vi "Stage Printing Loop.vi"(11 "Stage Actor.lvlib:Stage.lvclass":refnum<class "Stage.lvclass">) -> ()   [LabVIEW 2018, in "Stage Actor.lvlib" / "Stage.lvclass"]
uses:
  Stage.lvclass
  C:/Program Files (x86)/National Instruments/LabVIEW 2018/vi.lib/MGI/Panel Manager/Panel Actor/Panel Actor/Panel Actor.lvclass
  Stage.lvclass/Stage.ctl
  <instrlib>/Zaber A Series/Public/Action-Status/Streaming/Set Stream Speed and Acceleration (FW7).vi
  <instrlib>/Zaber A Series/Public/Action-Status/Streaming/Stream Line (FW7).vi
  <instrlib>/Zaber A Series/Zaber A Series.lvlib
  <vilib>/MGI/Panel Manager/Panel Actor/Panel Actor/Panel Actor.lvclass
panel:
  out "Stop":bool
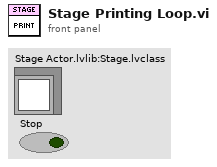
[diagram p1: front panel]
types:
  T1 = cluster{"Print Data":cluster{"XYZ":dbl[][], "Theta Phi":dbl[][], "Current Tool":i16[], "Speed":dbl[], "Feeder State":bool[]}, "Task":string}
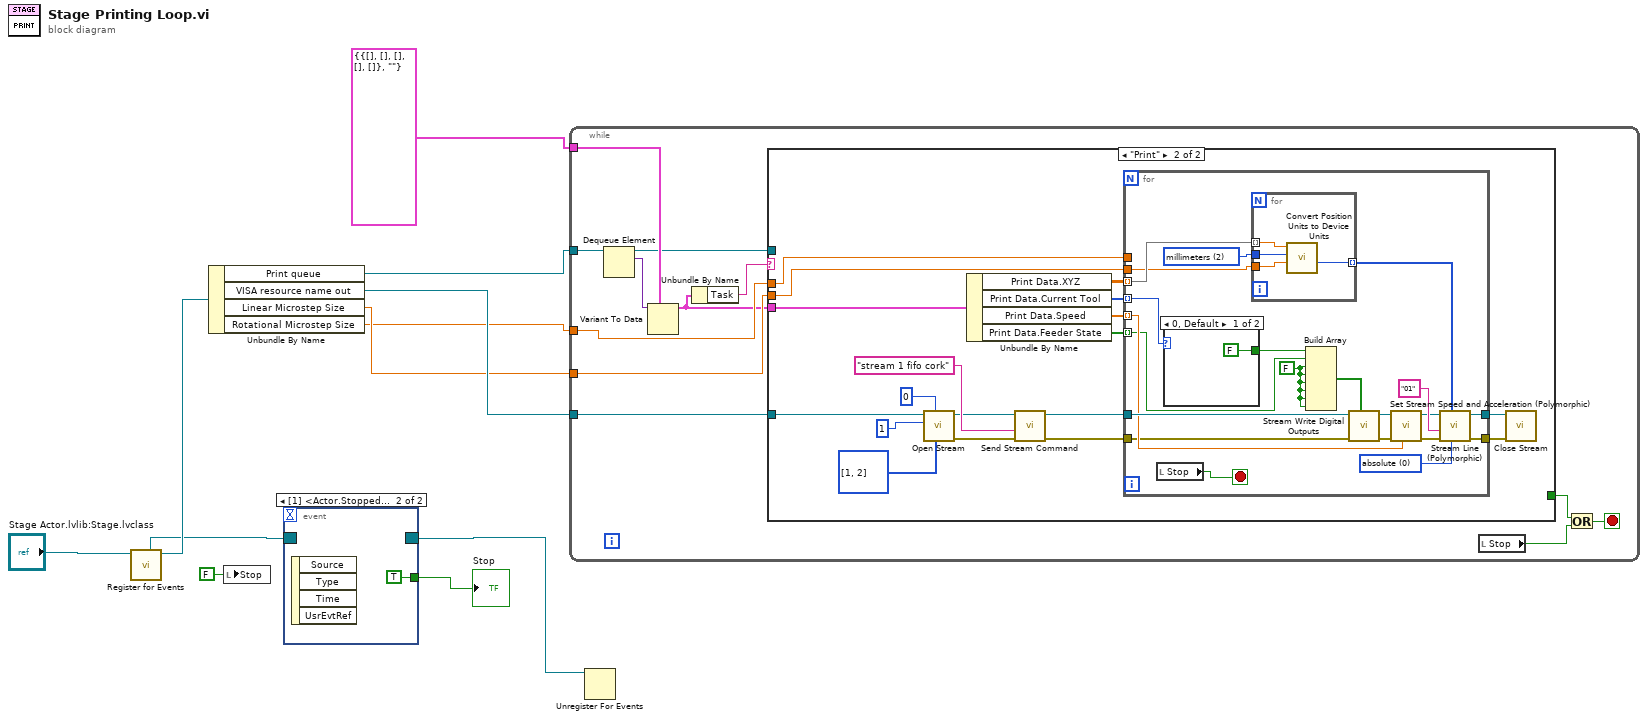
[diagram p0: block diagram]
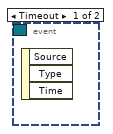
[diagram p2: hidden frame]
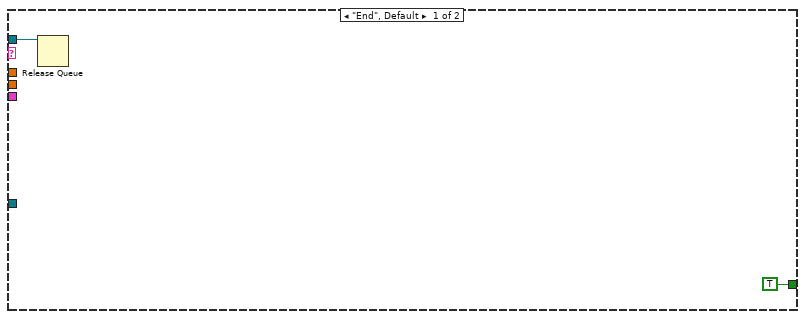
[diagram p3: hidden frame]
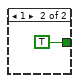
[diagram p4: hidden frame]
diagram:
  n1 = call <vilib>:"Register for Events.vi"("Panel Actor in"="Stage Actor.lvlib:Stage.lvclass") -> ("Panel Actor out"=w5:refnum<class "Stage.lvclass">, "Pnl Actor"=w4:refnum<event-registration>)  [unwired: 7 in, 2 out]
  n2 = Unbundle By Name(w5) -> ("Print queue"=w11:refnum<queue>, "VISA resource name out"=w10:refnum<visa-resource-name>, "Linear Microstep Size"=w9:dbl, "Rotational Microstep Size"=w8:dbl)
  n3 = local write "Stop"(FALSE ("Stop")) -> ()
  n4 = event shown="[1] <Actor.Stopped>: User Event" {
    selector: w4 -> [_ _]
    dyn-events: [_ _] -> w3
    timeout: _ -> [_ _]
    tunnel: [_ TRUE] -> w2
    event Timeout {
      n5 = event-data() -> ()  [unwired: 1 in, 3 out]
    }
    event User Event {
      n6 = event-data() -> ()  [unwired: 1 in, 4 out]
    }
  }
  "Stop" <- w2
  n7 = while {
    tunnel: w11 -> [w24]
    tunnel: w10 -> [w22]
    tunnel: w9 -> [w21]
    tunnel: w8 -> [w20]
    tunnel: T1 {"Print Data"={"XYZ"=[], "Theta Phi"=[], "Current Tool"=[], "Speed"=[], "Feeder State"=[]}, "Task"=""} ("Print Message") -> [w19]
    stop <- w16 stop-if-true
    n8 = Dequeue Element(queue=w24) -> (queue out=w14:refnum<queue>, element=w23:variant)  [unwired: 2 in, 2 out]
    n9 = Variant To Data(type=w19, Variant=w23) -> (data=w18:T1)  [unwired: 1 in, 1 out]
    n10 = Unbundle By Name(w18) -> ("Task"=w17:string)
    n11 = case shown="\"Print\"" w17 {
      tunnel: w18 -> [_ w44]
      tunnel: w22 -> [_ w33]
      tunnel: w21 -> [_ w31]
      tunnel: w20 -> [_ w29]
      tunnel: [TRUE _] -> w15
      tunnel: w14 -> [w25 _]
      frame "End", Default {
        n12 = Release Queue(queue=w25) -> ()  [unwired: 2 in, 3 out]
      }
      frame "Print" {
        n13 = call <instrlib>:"Open Stream.vi"("Axis Numbers (1,2)"=u8[] [1, 2], "Buffer Number (0)"=u8 0, "Stream Number (1)"=u8 1, "VISA resource name"=w33) -> ("error out"=w37:errorcluster, "VISA resource name out"=w38:refnum<visa-resource-name>)  [unwired: 6 in]
        n14 = Unbundle By Name(w44) -> ("Print Data.XYZ"=w43:dbl[][], "Print Data.Current Tool"=w42:i16[], "Print Data.Speed"=w41:dbl[], "Print Data.Feeder State"=w40:bool[])
        n15 = call <instrlib>:"Send Stream Command.vi"("error in (no error)"=w37, "Command"="stream 1 fifo cork", "VISA resource name"=w38) -> ("error out"=w28:errorcluster, "VISA resource name out"=w32:refnum<visa-resource-name>)  [unwired: 7 in]
        n16 = for {
          tunnel: w43 -> [w64] mode=indexing
          tunnel: w42 -> [w56] mode=indexing
          tunnel: w41 -> [w57] mode=indexing
          tunnel: w40 -> [w54] mode=indexing
          tunnel: w32 -> [w59]
          tunnel: w31 -> [w61]
          tunnel: [w51] -> w30
          tunnel: w29 -> [_]
          tunnel: w28 -> [w50]
          tunnel: [w47] -> w27
          stop <- w45 stop-if-true
          w52 = FALSE
          w62 = u16 2 items=["microsteps", "microns", "millimeters", "inches", "degrees"] ("Units (0: microsteps)")
          w65 = u16 0 items=["absolute", "relative"] ("Position Mode (0: absolute)")
          n17 = local read "Stop"() -> (w45:bool)
          n18 = case shown="0, Default" w56 {
            tunnel: [FALSE TRUE] -> w55
            frame 0, Default {
            }
            frame 1 {
            }
          }
          n19 = for {
            tunnel: w64 -> [w71] mode=indexing
            tunnel: [w70] -> w63 mode=indexing
            tunnel: w62 -> [w69]
            tunnel: w61 -> [w68]
            n20 = call <instrlib>:"Convert Position Units to Device Units.vi"("Microstep Size (0)"=w68, "Units (0: microsteps)"=w69, "Position (0)"=w71) -> ("Device Position (64-bit)"=w70:i64)  [unwired: 6 in, 2 out]
          }
          n21 = Build Array(w55, w54, w52, w52, w52, w52, w52, w52) -> (w53:bool[])
          n22 = call <instrlib>:"Stream Write Digital Outputs.vi"("Digital Outputs"=w53, "error in (no error)"=w50, "VISA resource name"=w59) -> ("error out"=w49:errorcluster, "VISA resource name out"=w58:refnum<visa-resource-name>)  [unwired: 7 in]
          n23 = call-poly <instrlib>:"Set Stream Speed and Acceleration (Polymorphic).vi"("Maximum Speed (0)"=w57, "error in (no error)"=w49, "VISA resource name"=w58) -> ("error out"=w48:errorcluster, "VISA resource name out"=w46:refnum<visa-resource-name>)  [unwired: 7 in]
          n24 = call-poly <instrlib>:"Stream Line (Polymorphic).vi"("Position Mode (0: absolute)"=w65, "Coordinates"=w63, "error in (no error)"=w48, "Device Number"="01", "VISA resource name"=w46) -> ("error out"=w47:errorcluster, "VISA resource name out"=w51:refnum<visa-resource-name>)  [unwired: 5 in]
        }
        n25 = call <instrlib>:"Close Stream.vi"("error in (no error)"=w27, "VISA resource name"=w30) -> ()  [unwired: 8 in, 2 out]
      }
    }
    n26 = local read "Stop"() -> (w13:bool)
    n27 = Or(x=w15, y=w13) -> (x .or. y?=w16:bool)
  }
  n28 = Unregister For Events(event registration refnum=w3) -> ()  [unwired: 1 in, 1 out]
